vi "respond JSON.vi"(11 "Message In":cluster{"Message":string[], "Data In":T1}={"Message"=[], "Data In"={"UI References"={"Exit Ref"=refnum, "Save Ref"=refnum, "Open Ref"=refnum, "Export Ref"=refnum, "Acquire Ref"=refnum, "Configure Ref"=refnum, "Graph Ref"=refnum, "Clear Ref"=refnum, "Analyze Ref"=refnum, "Status Ref"=refnum, "Snapshot Ref"=refnum}, "User Specified"={"Hardware Configuration"={"Signal Channel"="", "Response Channel"="", "Trigger Channel"="", "Number of Acquisitions"=0.0}, "Analysis Configuration"={"Statistics"=TRUE}, "Signal Type"=enum."Single Chirp", "New Data Behavior"=enum."Replace", "Signal Configuration"={"Chirp Amplitude"=0.1, "I/O Limit"=10.0, "Sample Rate"=1000000.0, "Chirp Duration (s)"=0.01, "Upper Frequency"=0.0, "Lower Frequency"=0.0, "Windowing"=enum."None"}, "Waveform File"="", "Save Location"=""}}}) -> ()   [LabVIEW 2017]
uses:
  controls/Data.ctl
  controls/UI References.ctl
  controls/User Specified Data.ctl
  controls/HW Configuration.ctl
  controls/Analysis Configuration.ctl
  controls/New Data Behavior.ctl
  controls/Signal Configuration.ctl
  <resource>/objmgr/daqmx.rc
panel:
  out "length":i32
  out "JSON string":string
  out "Data Out":T1={"UI References"={"Exit Ref"=refnum, "Save Ref"=refnum, "Open Ref"=refnum, "Export Ref"=refnum, "Acquire Ref"=refnum, "Configure Ref"=refnum, "Graph Ref"=refnum, "Clear Ref"=refnum, "Analyze Ref"=refnum, "Status Ref"=refnum, "Snapshot Ref"=refnum}, "User Specified"={"Hardware Configuration"={"Signal Channel"="", "Response Channel"="", "Trigger Channel"="", "Number of Acquisitions"=0.0}, "Analysis Configuration"={"Statistics"=TRUE}, "Signal Type"=enum."Single Chirp", "New Data Behavior"=enum."Replace", "Signal Configuration"={"Chirp Amplitude"=0.1, "I/O Limit"=10.0, "Sample Rate"=1000000.0, "Chirp Duration (s)"=0.01, "Upper Frequency"=0.0, "Lower Frequency"=0.0, "Windowing"=enum."None"}, "Waveform File"="", "Save Location"=""}}
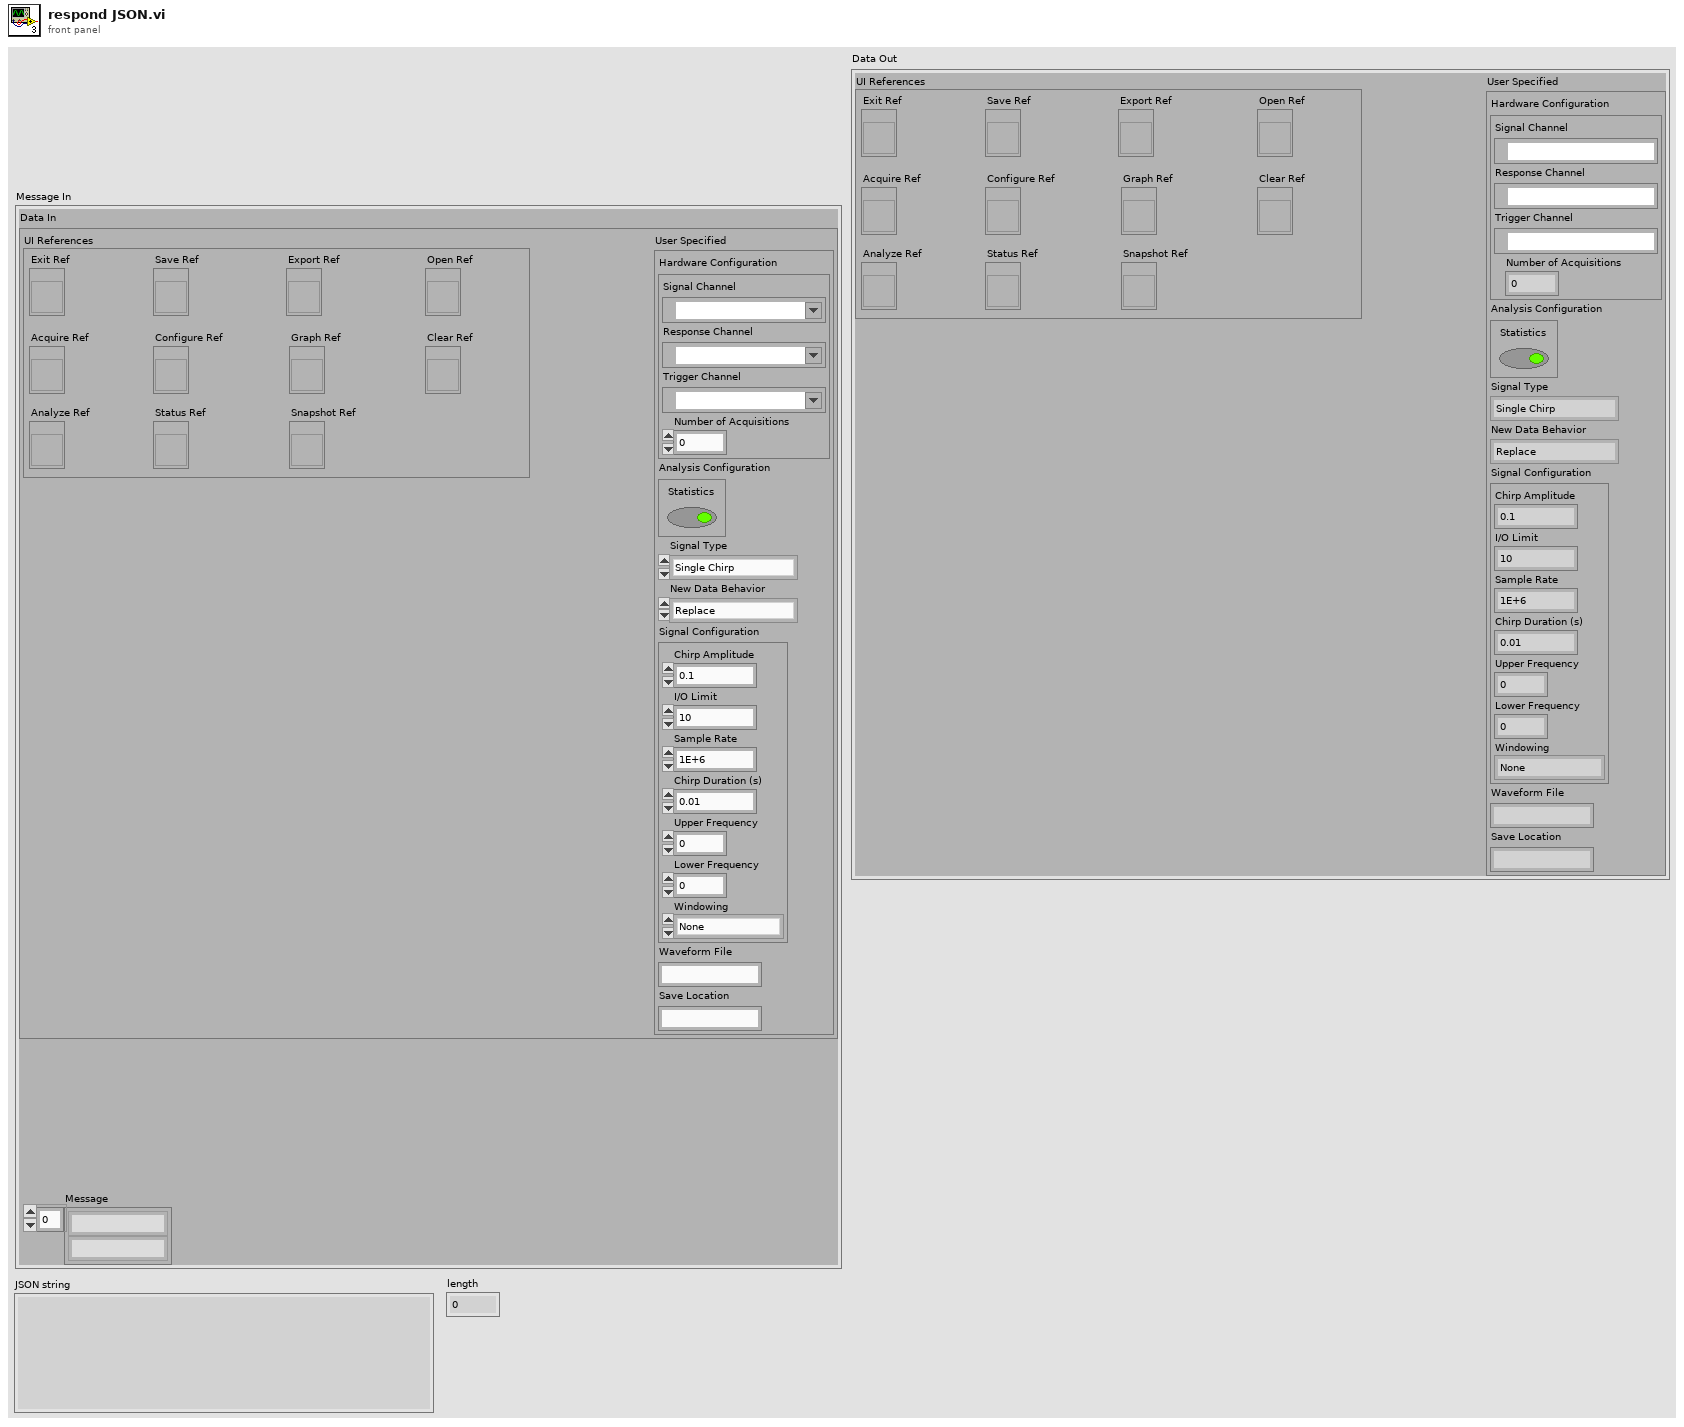
[diagram p1: front panel]
types:
  T1 = typedef "Data.ctl" = cluster{"UI References":T2, "User Specified":T3}
  T2 = typedef "UI References.ctl" = cluster{"Exit Ref":refnum<vi>, "Save Ref":refnum<vi>, "Open Ref":refnum<vi>, "Export Ref":refnum<vi>, "Acquire Ref":refnum<vi>, "Configure Ref":refnum<vi>, "Graph Ref":refnum<vi>, "Clear Ref":refnum<vi>, "Analyze Ref":refnum<vi>, "Status Ref":refnum<vi>, "Snapshot Ref":refnum<vi>}
  T3 = typedef "User Specified Data.ctl" = cluster{"Hardware Configuration":T4, "Analysis Configuration":T5, "Signal Type":enum16{"Single Chirp", "From Excel"}, "New Data Behavior":T6, "Signal Configuration":T7, "Waveform File":string, "Save Location":string}
  T4 = typedef "HW Configuration.ctl" = cluster{"Signal Channel":tag, "Response Channel":tag, "Trigger Channel":tag, "Number of Acquisitions":dbl}
  T5 = typedef "Analysis Configuration.ctl" = cluster{"Statistics":bool}
  T6 = typedef "New Data Behavior.ctl" = enum16{"Replace", "Overlay", "Append"}
  T7 = typedef "Signal Configuration.ctl" = cluster{"Chirp Amplitude":dbl, "I/O Limit":dbl, "Sample Rate":dbl, "Chirp Duration (s)":dbl, "Upper Frequency":dbl, "Lower Frequency":dbl, "Windowing":enum16{"None", "Exponential", "Flat top", "Hamming", "Hanning", "Kaiser-Bessel", "Rectangular"}}
  T8 = cluster{"message_name":string, "signalChannels":string[]}
  T9 = cluster{"message_name":string, "param_name":string, "param_value":string}
  T10 = enum16{"None", "Exponential", "Flat top", "Hamming", "Hanning", "Kaiser-Bessel", "Rectangular"}
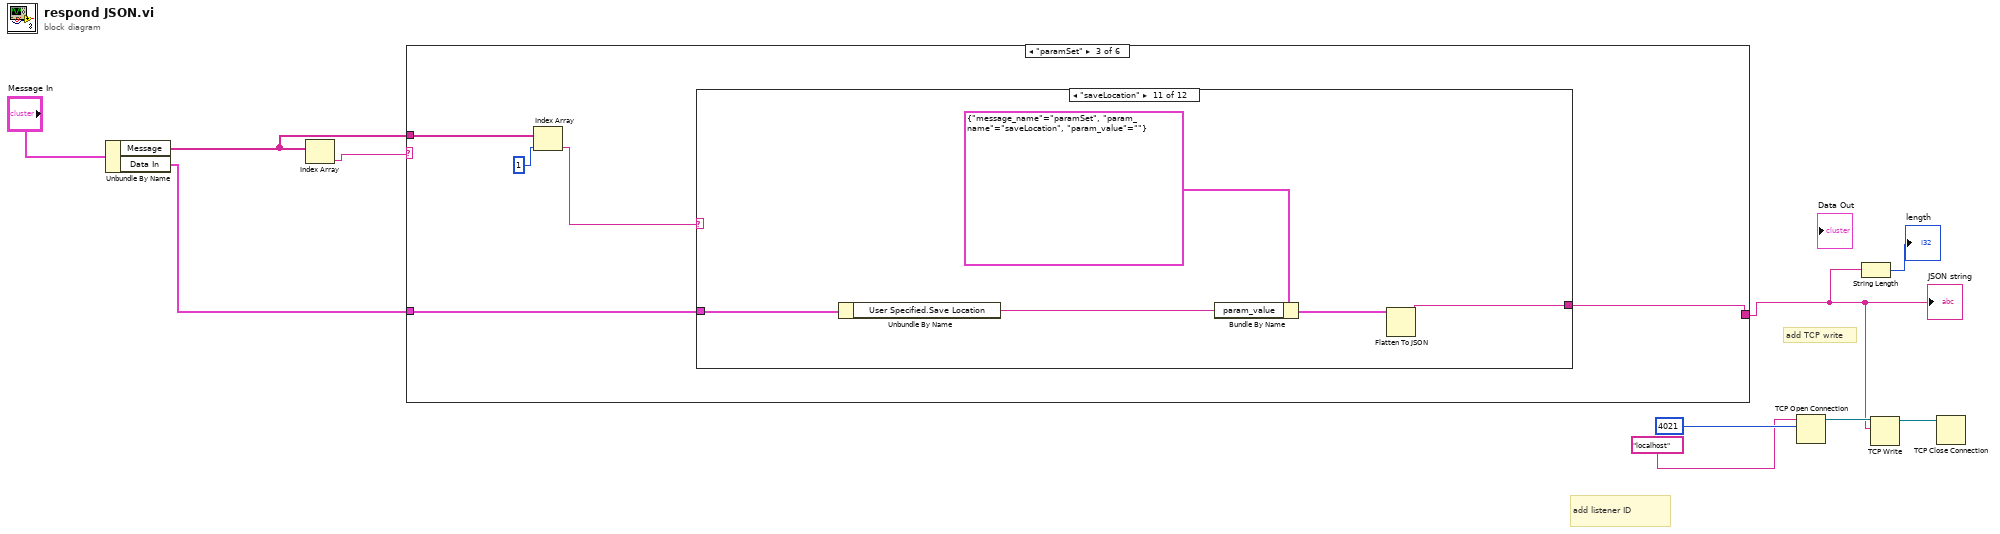
[diagram p0: block diagram]
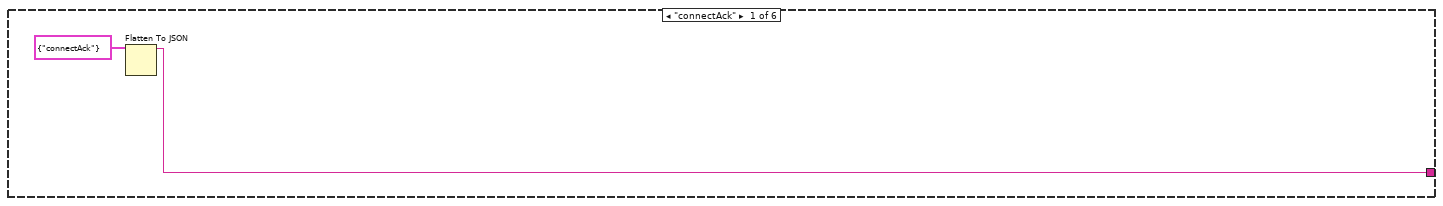
[diagram p2: hidden frame]
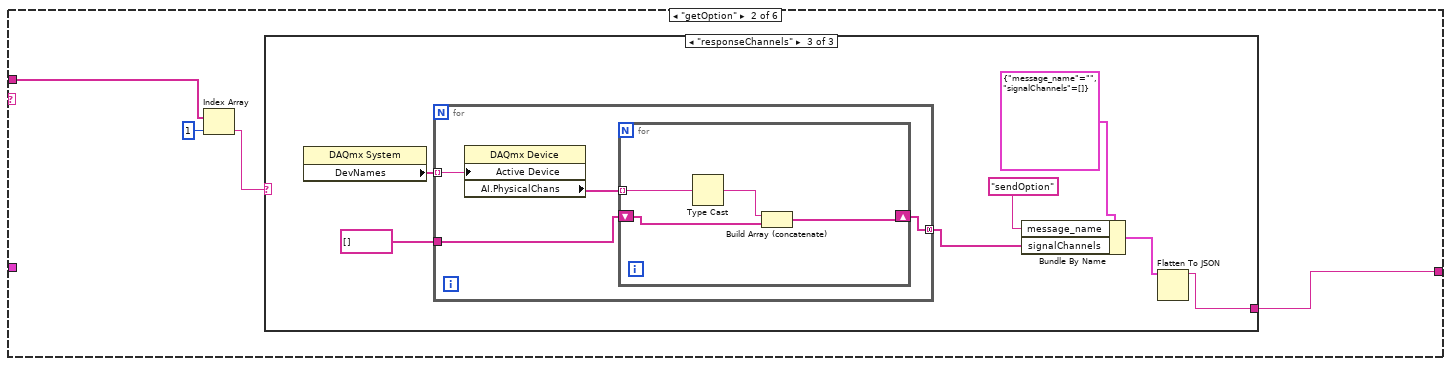
[diagram p3: hidden frame]
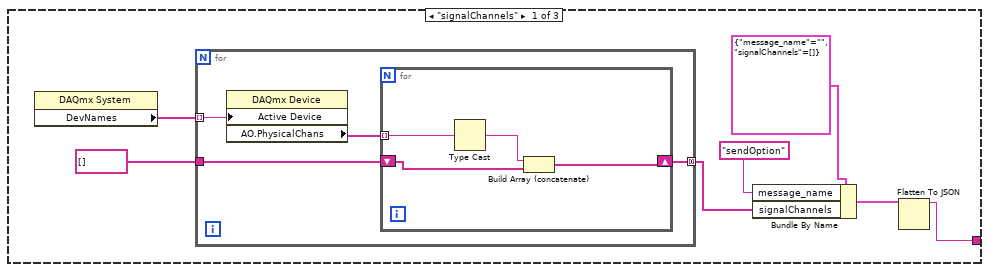
[diagram p4: hidden frame]
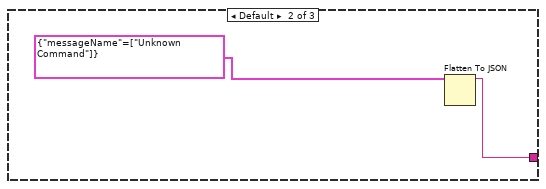
[diagram p5: hidden frame]
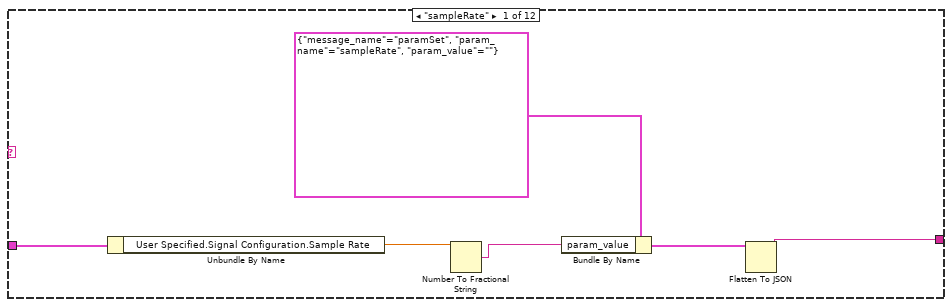
[diagram p6: hidden frame]
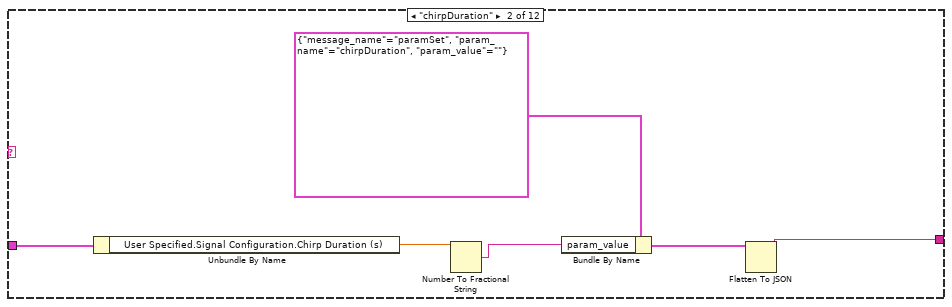
[diagram p7: hidden frame]
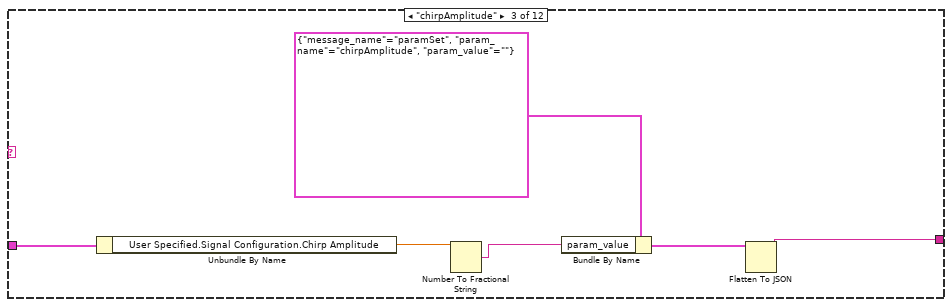
[diagram p8: hidden frame]
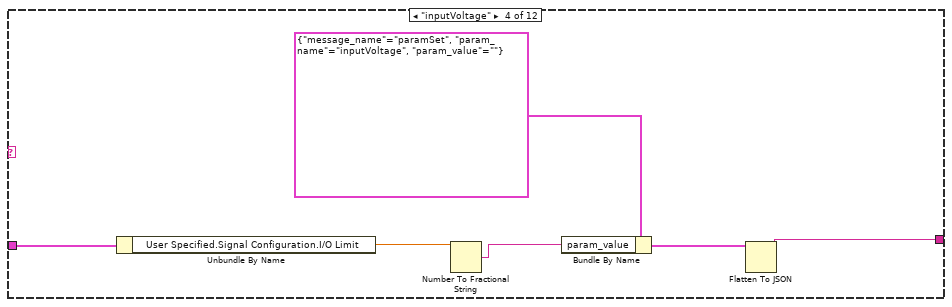
[diagram p9: hidden frame]
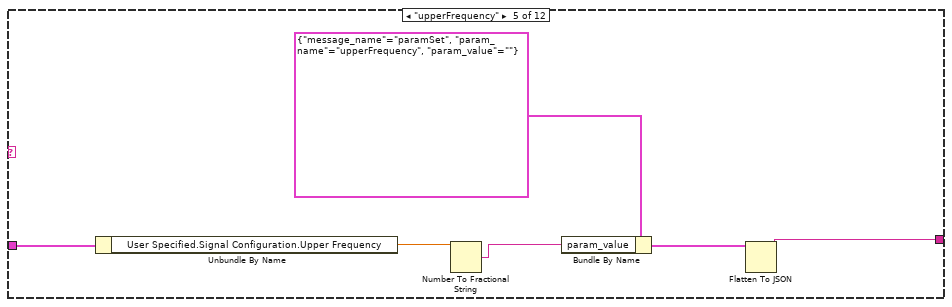
[diagram p10: hidden frame]
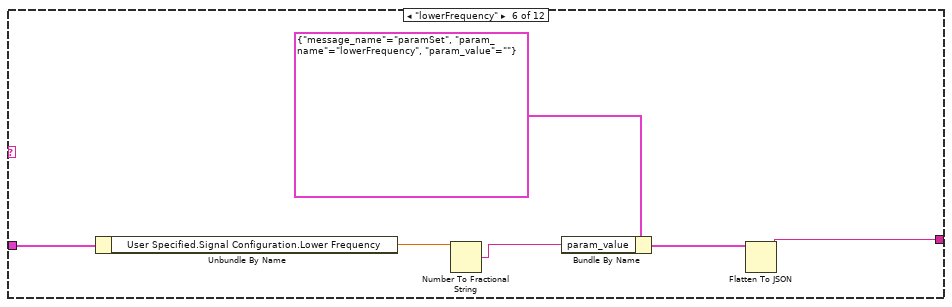
[diagram p11: hidden frame]
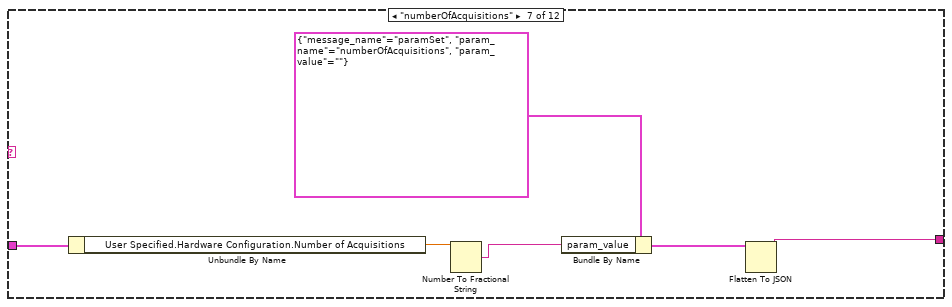
[diagram p12: hidden frame]
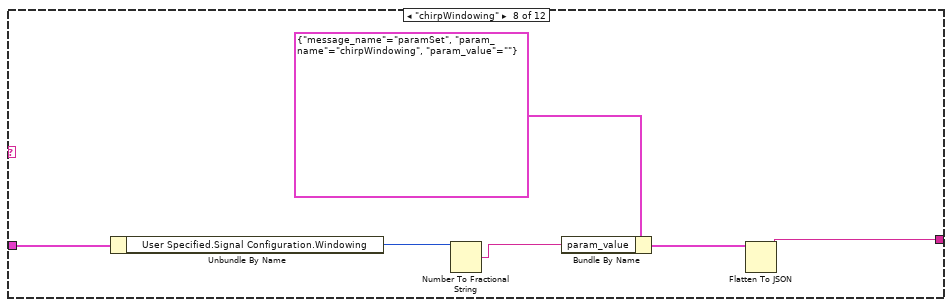
[diagram p13: hidden frame]
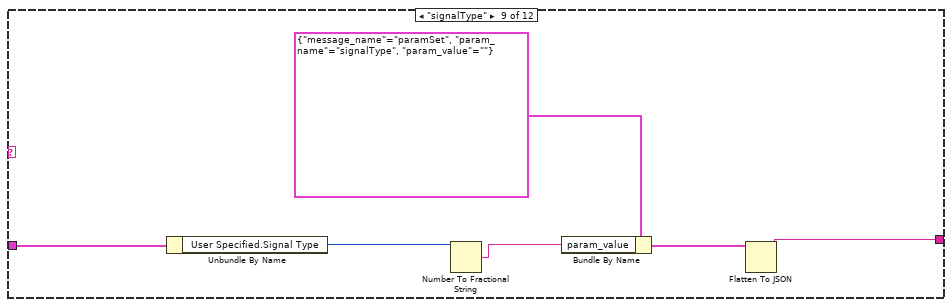
[diagram p14: hidden frame]
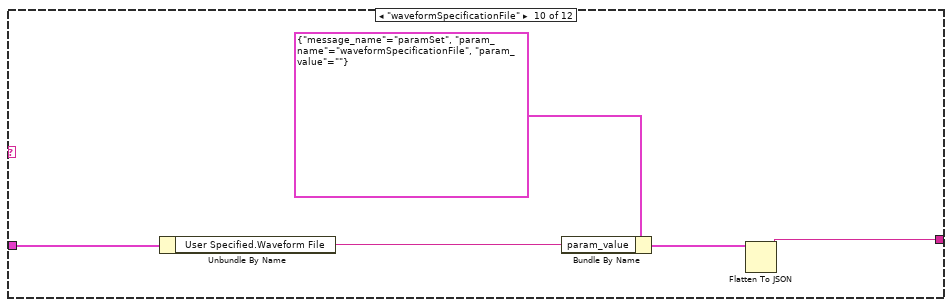
[diagram p15: hidden frame]
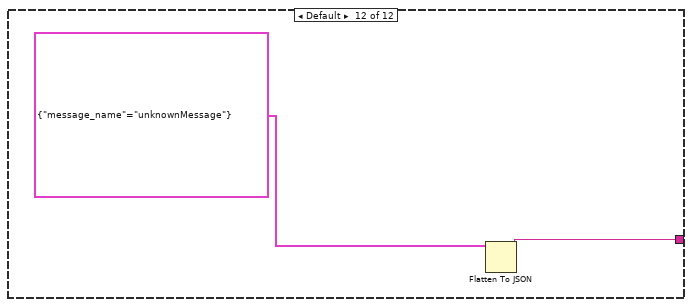
[diagram p16: hidden frame]
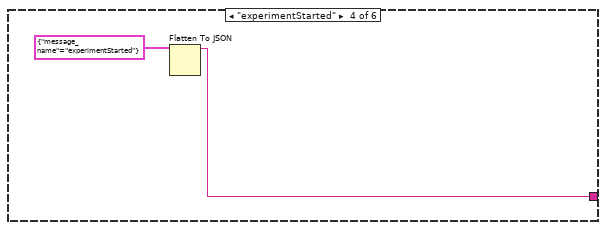
[diagram p17: hidden frame]
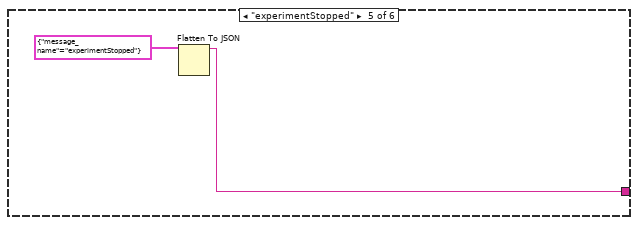
[diagram p18: hidden frame]
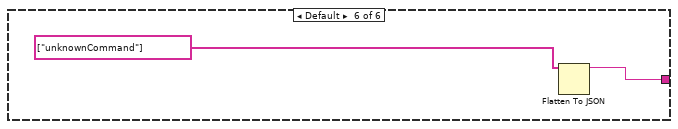
[diagram p19: hidden frame]
diagram:
  # "add TCP write"
  # "add listener ID"
  n1 = Unbundle By Name("Message In") -> ("Message"=w8:string[], "Data In"=w7:T1)
  n2 = Index Array(array=w8) -> (element=w9:string)  [unwired: 1 in]
  n3 = case shown="\"paramSet\"" w9 {
    tunnel: [w11 w15 w53 w120 w122 w125] -> w2
    tunnel: w8 -> [_ w14 w51 _ _ _]
    tunnel: w7 -> [_ _ w49 _ _ _]
    frame "connectAck" {
      n4 = Flatten To JSON(anything=cluster{"message_name":string} {"message_name"="connectAck"}) -> (JSON string=w11:string)  [unwired: 2 in, 1 out]
    }
    frame "getOption" {
      n5 = Index Array(array=w14, index=1) -> (element=w13:string)
      n6 = case shown="\"responseChannels\"" w13 {
        tunnel: [w21 w33 w38] -> w15
        frame "signalChannels" {
          n7 = property class="DAQmx System"() -> ("DevNames"=w23:tag[])  [unwired: 2 in, 2 out]
          n8 = for {
            tunnel: w23 -> [w27] mode=indexing
            tunnel: string[] [] ("signalChannels") -> [w26]
            tunnel: [w24] -> w17 mode=concatenating
            n9 = property class="DAQmx Device"("Active Device"=w27) -> ("AO.PhysicalChans"=w25:tag[])  [unwired: 2 in, 2 out]
            n10 = for {
              shift-right: [w31] -> w24
              shift-left: w26 -> [w30]
              tunnel: w25 -> [w28] mode=indexing
              n11 = Type Cast(x=w28) -> (*(type *) &x=w29:string)  [unwired: 1 in]
              n12 = Build Array (concatenate)(w29, w30) -> (w31:string[])
            }
          }
          n13 = Bundle By Name(cluster=T8 {"message_name"="", "signalChannels"=[]} ("signalChannels"), "message_name"="sendOption", "signalChannels"=w17) -> (w19:T8)
          n14 = Flatten To JSON(anything=w19) -> (JSON string=w21:string)  [unwired: 2 in, 1 out]
        }
        frame Default {
          n15 = Flatten To JSON(anything=cluster{"messageName":string[]} {"messageName"=["Unknown Command"]} ("message_name")) -> (JSON string=w33:string)  [unwired: 2 in, 1 out]
        }
        frame "responseChannels" {
          n16 = property class="DAQmx System"() -> ("DevNames"=w40:tag[])  [unwired: 2 in, 2 out]
          n17 = for {
            tunnel: w40 -> [w44] mode=indexing
            tunnel: string[] [] ("deWae") -> [w42]
            tunnel: [w41] -> w35 mode=concatenating
            n18 = property class="DAQmx Device"("Active Device"=w44) -> ("AI.PhysicalChans"=w43:tag[])  [unwired: 2 in, 2 out]
            n19 = for {
              shift-right: [w45] -> w41
              shift-left: w42 -> [w46]
              tunnel: w43 -> [w47] mode=indexing
              n20 = Type Cast(x=w47) -> (*(type *) &x=w48:string)  [unwired: 1 in]
              n21 = Build Array (concatenate)(w48, w46) -> (w45:string[])
            }
          }
          n22 = Bundle By Name(cluster=T8 {"message_name"="", "signalChannels"=[]} ("signalChannels"), "message_name"="sendOption", "signalChannels"=w35) -> (w34:T8)
          n23 = Flatten To JSON(anything=w34) -> (JSON string=w38:string)  [unwired: 2 in, 1 out]
        }
      }
    }
    frame "paramSet" {
      n24 = Index Array(array=w51, index=1) -> (element=w50:string)
      n25 = case shown="\"saveLocation\"" w50 {
        tunnel: [w59 w65 w71 w77 w83 w89 w95 w101 w107 w112 w117 w119] -> w53
        tunnel: w49 -> [w56 w62 w68 w74 w80 w86 w92 w98 w104 w109 w114 _]
        frame "sampleRate" {
          n26 = Unbundle By Name(w56) -> ("User Specified.Signal Configuration.Sample Rate"=w55:dbl)
          n27 = Number To Fractional String(number=w55) -> (F-format string=w54:string)  [unwired: 3 in]
          n28 = Bundle By Name(cluster=T9 {"message_name"="paramSet", "param_name"="sampleRate", "param_value"=""}, "param_value"=w54) -> (w57:T9)
          n29 = Flatten To JSON(anything=w57) -> (JSON string=w59:string)  [unwired: 2 in, 1 out]
        }
        frame "chirpDuration" {
          n30 = Unbundle By Name(w62) -> ("User Specified.Signal Configuration.Chirp Duration (s)"=w61:dbl)
          n31 = Number To Fractional String(number=w61) -> (F-format string=w60:string)  [unwired: 3 in]
          n32 = Bundle By Name(cluster=T9 {"message_name"="paramSet", "param_name"="chirpDuration", "param_value"=""}, "param_value"=w60) -> (w63:T9)
          n33 = Flatten To JSON(anything=w63) -> (JSON string=w65:string)  [unwired: 2 in, 1 out]
        }
        frame "chirpAmplitude" {
          n34 = Unbundle By Name(w68) -> ("User Specified.Signal Configuration.Chirp Amplitude"=w67:dbl)
          n35 = Number To Fractional String(number=w67) -> (F-format string=w66:string)  [unwired: 3 in]
          n36 = Bundle By Name(cluster=T9 {"message_name"="paramSet", "param_name"="chirpAmplitude", "param_value"=""}, "param_value"=w66) -> (w69:T9)
          n37 = Flatten To JSON(anything=w69) -> (JSON string=w71:string)  [unwired: 2 in, 1 out]
        }
        frame "inputVoltage" {
          n38 = Unbundle By Name(w74) -> ("User Specified.Signal Configuration.I/O Limit"=w73:dbl)
          n39 = Number To Fractional String(number=w73) -> (F-format string=w72:string)  [unwired: 3 in]
          n40 = Bundle By Name(cluster=T9 {"message_name"="paramSet", "param_name"="inputVoltage", "param_value"=""}, "param_value"=w72) -> (w75:T9)
          n41 = Flatten To JSON(anything=w75) -> (JSON string=w77:string)  [unwired: 2 in, 1 out]
        }
        frame "upperFrequency" {
          n42 = Unbundle By Name(w80) -> ("User Specified.Signal Configuration.Upper Frequency"=w79:dbl)
          n43 = Number To Fractional String(number=w79) -> (F-format string=w78:string)  [unwired: 3 in]
          n44 = Bundle By Name(cluster=T9 {"message_name"="paramSet", "param_name"="upperFrequency", "param_value"=""}, "param_value"=w78) -> (w81:T9)
          n45 = Flatten To JSON(anything=w81) -> (JSON string=w83:string)  [unwired: 2 in, 1 out]
        }
        frame "lowerFrequency" {
          n46 = Unbundle By Name(w86) -> ("User Specified.Signal Configuration.Lower Frequency"=w85:dbl)
          n47 = Number To Fractional String(number=w85) -> (F-format string=w84:string)  [unwired: 3 in]
          n48 = Bundle By Name(cluster=T9 {"message_name"="paramSet", "param_name"="lowerFrequency", "param_value"=""}, "param_value"=w84) -> (w87:T9)
          n49 = Flatten To JSON(anything=w87) -> (JSON string=w89:string)  [unwired: 2 in, 1 out]
        }
        frame "numberOfAcquisitions" {
          n50 = Unbundle By Name(w92) -> ("User Specified.Hardware Configuration.Number of Acquisitions"=w91:dbl)
          n51 = Number To Fractional String(number=w91) -> (F-format string=w90:string)  [unwired: 3 in]
          n52 = Bundle By Name(cluster=T9 {"message_name"="paramSet", "param_name"="numberOfAcquisitions", "param_value"=""}, "param_value"=w90) -> (w93:T9)
          n53 = Flatten To JSON(anything=w93) -> (JSON string=w95:string)  [unwired: 2 in, 1 out]
        }
        frame "chirpWindowing" {
          n54 = Unbundle By Name(w98) -> ("User Specified.Signal Configuration.Windowing"=w97:T10)
          n55 = Number To Fractional String(number=w97) -> (F-format string=w96:string)  [unwired: 3 in]
          n56 = Bundle By Name(cluster=T9 {"message_name"="paramSet", "param_name"="chirpWindowing", "param_value"=""}, "param_value"=w96) -> (w99:T9)
          n57 = Flatten To JSON(anything=w99) -> (JSON string=w101:string)  [unwired: 2 in, 1 out]
        }
        frame "signalType" {
          n58 = Unbundle By Name(w104) -> ("User Specified.Signal Type"=w103:enum16{"Single Chirp", "From Excel"})
          n59 = Number To Fractional String(number=w103) -> (F-format string=w102:string)  [unwired: 3 in]
          n60 = Bundle By Name(cluster=T9 {"message_name"="paramSet", "param_name"="signalType", "param_value"=""}, "param_value"=w102) -> (w105:T9)
          n61 = Flatten To JSON(anything=w105) -> (JSON string=w107:string)  [unwired: 2 in, 1 out]
        }
        frame "waveformSpecificationFile" {
          n62 = Unbundle By Name(w109) -> ("User Specified.Waveform File"=w108:string)
          n63 = Bundle By Name(cluster=T9 {"message_name"="paramSet", "param_name"="waveformSpecificationFile", "param_value"=""}, "param_value"=w108) -> (w110:T9)
          n64 = Flatten To JSON(anything=w110) -> (JSON string=w112:string)  [unwired: 2 in, 1 out]
        }
        frame "saveLocation" {
          n65 = Unbundle By Name(w114) -> ("User Specified.Save Location"=w113:string)
          n66 = Bundle By Name(cluster=T9 {"message_name"="paramSet", "param_name"="saveLocation", "param_value"=""}, "param_value"=w113) -> (w115:T9)
          n67 = Flatten To JSON(anything=w115) -> (JSON string=w117:string)  [unwired: 2 in, 1 out]
        }
        frame Default {
          n68 = Flatten To JSON(anything=cluster{"message_name":string} {"message_name"="unknownMessage"}) -> (JSON string=w119:string)  [unwired: 2 in, 1 out]
        }
      }
    }
    frame "experimentStarted" {
      n69 = Flatten To JSON(anything=cluster{"message_name":string} {"message_name"="experimentStarted"}) -> (JSON string=w120:string)  [unwired: 2 in, 1 out]
    }
    frame "experimentStopped" {
      n70 = Flatten To JSON(anything=cluster{"message_name":string} {"message_name"="experimentStopped"}) -> (JSON string=w122:string)  [unwired: 2 in, 1 out]
    }
    frame Default {
      n71 = Flatten To JSON(anything=string[] ["unknownCommand"]) -> (JSON string=w125:string)  [unwired: 2 in, 1 out]
    }
  }
  "JSON string" <- w2
  n72 = TCP Open Connection(address="localhost", remote port or service name=u16 4021) -> (connection ID=w4:refnum<k5>)  [unwired: 3 in, 1 out]
  n73 = String Length(string=w2) -> (length=→"length":i32)
  n74 = TCP Write(connection ID=w4, data in=w2) -> (connection ID out=w3:refnum<k5>)  [unwired: 2 in, 2 out]
  n75 = TCP Close Connection(connection ID=w3) -> ()  [unwired: 2 in, 2 out]
